vi "mult_process - копия.vi"() -> ()   [LabVIEW 2013]
uses:
  G:/Romanova/results_cluster.ctl
  <vilib>/Utility/file.llb/Read From Spreadsheet File (DBL).vi
  <vilib>/gmath/statdist.llb/Student t Inverse CDF.vi
  <vilib>/Analysis/NI_AALBase.lvlib
  <vilib>/gmath/NI_Gmath.lvlib
panel:
  in  "Строка форматирования":string="%_5f ± %_3f; %_2f"
  out "Результат измерений":string
  in  "Pдов":dbl=0.95
  in  "Границы НСП":dbl
  out "Результаты обработки":T1 {"Dдов рез" format="%#.4g"; "S сумм" format="%#.4g"; "К" format="%#.4g"; "Dдов случ." format="%#.4g"; "Sхср" format="%#.4g"; "S" format="%#.4g"}
  in  "Записать результат":bool
  in  "Получить данные":bool
  in  "Вычислить Dдов":bool
  out "Ряд измерений":dbl[](graph)
  in  "Стоп":bool
  in  "Вычислить оценки":bool
  in  "Путь":path caption="Путь к файлу"
  # "Обработка результатов многократных измерений"
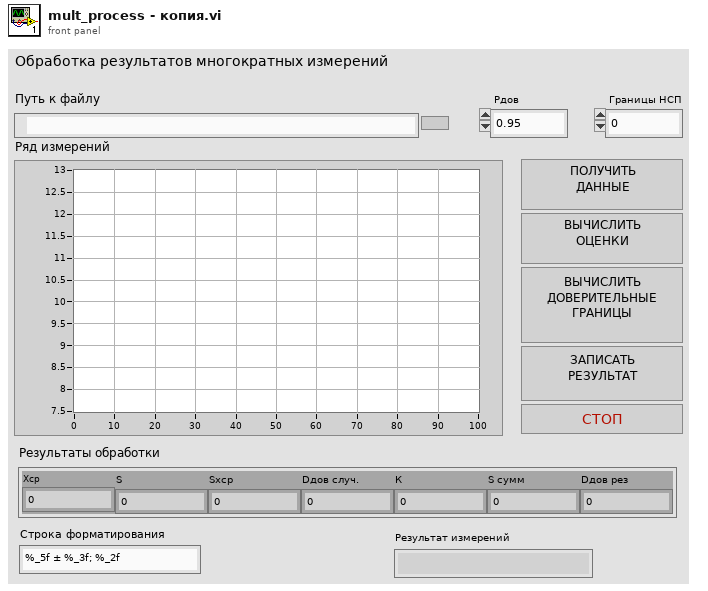
[diagram p1: front panel]
types:
  T1 = typedef "results_cluster.ctl" = cluster{"Xср":dbl, "S":dbl, "Sхср":dbl, "Dдов случ.":dbl, "К":dbl, "S сумм":dbl, "Dдов рез":dbl}
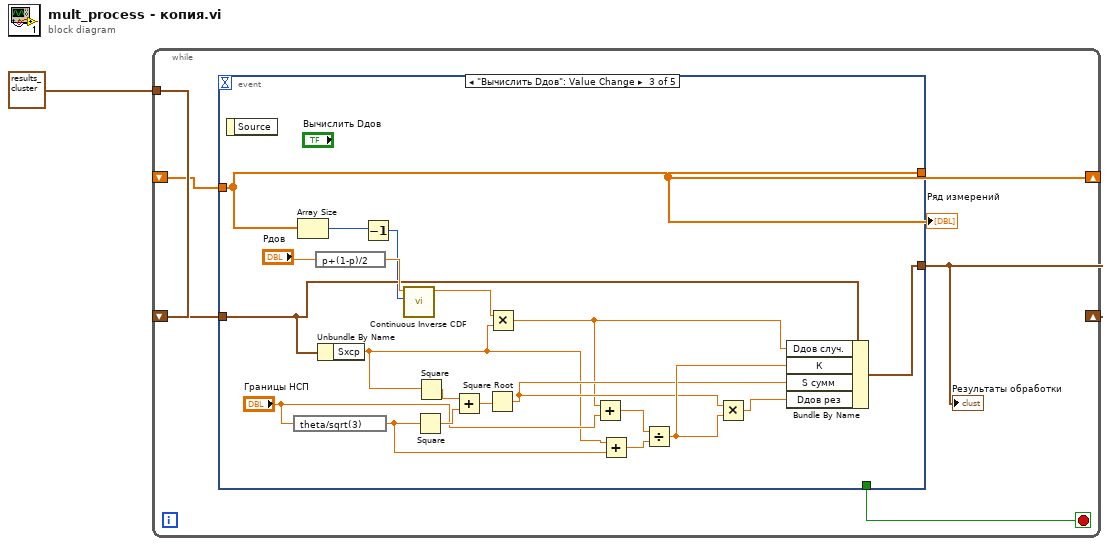
[diagram p0: block diagram]
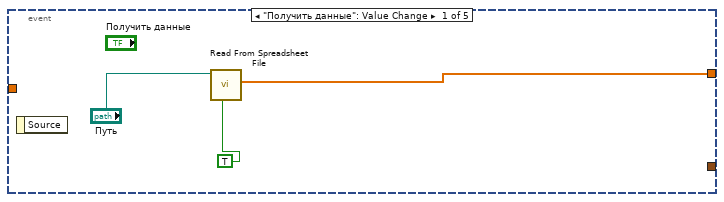
[diagram p2: hidden frame]
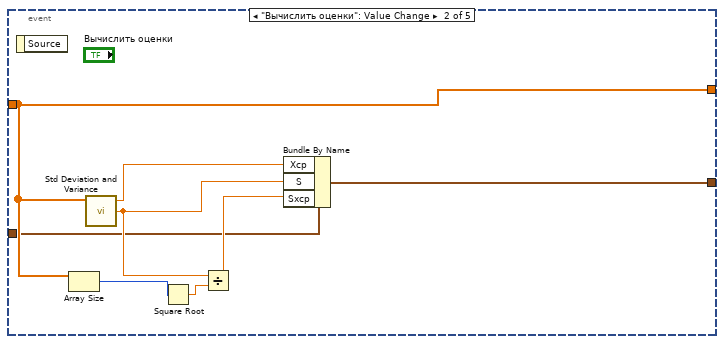
[diagram p3: hidden frame]
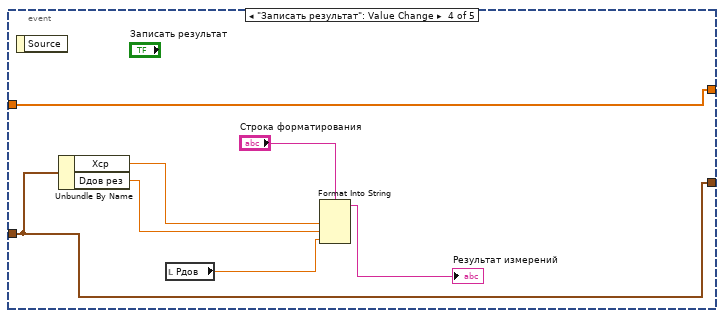
[diagram p4: hidden frame]
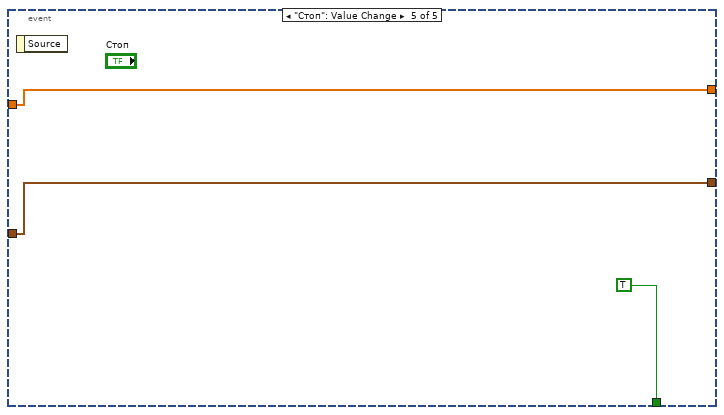
[diagram p5: hidden frame]
diagram:
  w1 = T1 {"Xср"=1.3199999999999998, "S"=0.130384048104053, "Sхср"=0.05830951894845301, "Dдов случ."=0.16189317847087023, "К"=2.43060784036949, "S сумм"=0.06506407098647712, "Dдов рез"=0.15814524106608838} ("Результаты обработки")
  n1 = while {
    shift-right: [w6] -> _
    shift-left: _ -> [w5]
    shift-right: [w3] -> _
    shift-left: w1 -> [w4]
    tunnel: w1 -> [_]
    stop <- w2 stop-if-true
    n2 = event shown="[2] \"Вычислить Dдов\": Value Change" {
      selector: _ -> [_ _ _ _ _]
      dyn-events: _ -> [_ _ _ _ _]
      timeout: _ -> [_ _ _ _ _]
      tunnel: [w7 w15 w20 w38 w47] -> w6
      tunnel: w5 -> [_ w15 w20 w38 w47]
      tunnel: w4 -> [_ w10 w22 w44 w46]
      tunnel: [_ w16 w35 w44 w46] -> w3
      tunnel: [_ _ _ _ TRUE] -> w2
      event "Получить данные": Value Change {
        n3 = event-data() -> ()  [unwired: 1 in, 1 out]
        n4 = call-poly <vilib>:"Read From Spreadsheet File.vi"("transpose (no:F)"=TRUE, "file path (dialog if empty)"="Путь") -> ("first row"=w7:dbl[])  [unwired: 5 in, 4 out]
      }
      event "Вычислить оценки": Value Change {
        n5 = event-data() -> ()  [unwired: 1 in, 1 out]
        n6 = Array Size(array=w15) -> (size(s)=w14:i32)
        n7 = call <vilib>:"Std Deviation and Variance.vi"("X"=w15) -> ("mean"=w17:dbl, "standard deviation"=w12:dbl)  [unwired: 1 in, 1 out]
        n8 = Square Root(x=w14) -> (sqrt(x)=w13:dbl)
        n9 = Divide(x=w12, y=w13) -> (x/y=w11:dbl)
        n10 = Bundle By Name(cluster=w10, "Xср"=w17, "S"=w12, "Sхср"=w11) -> (w16:T1)
      }
      event "Вычислить Dдов": Value Change {
        n11 = event-data() -> ()  [unwired: 1 in, 1 out]
        n12 = expression code="theta/sqrt(3)"("Границы НСП") -> (w23:dbl)
        n13 = Array Size(array=w20) -> (size(s)=w19:i32)
        n14 = expression code="p+(1-p)/2"("Pдов") -> (w36:dbl)
        n15 = Unbundle By Name(w22) -> ("Sхср"=w21:dbl)
        n16 = Decrement(x=w19) -> (x-1=w18:i32)
        n17 = call-poly <vilib>:"Continuous Inverse CDF.vi"("k degrees of freedom"=w18, "cdf(x)"=w36) -> ("x"=w31:dbl)  [unwired: 8 in, 1 out]
        n18 = Square(x=w23) -> (x^2=w33:dbl)
        n19 = Square(x=w21) -> (x^2=w34:dbl)
        n20 = Add(x=w34, y=w33) -> (x+y=w32:dbl)
        n21 = Square Root(x=w32) -> (sqrt(x)=w27:dbl)
        n22 = Multiply(x=w31, y=w21) -> (x*y=w25:dbl)
        n23 = Add(x=w25, y="Границы НСП") -> (x+y=w30:dbl)
        n24 = Add(x=w21, y=w23) -> (x+y=w29:dbl)
        n25 = Divide(x=w30, y=w29) -> (x/y=w28:dbl)
        n26 = Multiply(x=w27, y=w28) -> (x*y=w26:dbl)
        n27 = Bundle By Name(cluster=w22, "Dдов случ."=w25, "К"=w28, "S сумм"=w27, "Dдов рез"=w26) -> (w35:T1)
      }
      event "Записать результат": Value Change {
        n28 = event-data() -> ()  [unwired: 1 in, 1 out]
        n29 = Unbundle By Name(w44) -> ("Xср"=w39:dbl, "Dдов рез"=w40:dbl)
        n30 = local read "Pдов"() -> (w41:dbl)
        n31 = Format Into String(format string="Строка форматирования", w39, w40, w41) -> (resulting string=→"Результат измерений":string)  [unwired: 2 in, 1 out]
      }
      event "Стоп": Value Change {
        n32 = event-data() -> ()  [unwired: 1 in, 1 out]
      }
    }
    "Ряд измерений" <- w6
    "Результаты обработки" <- w3
  }
